vi "Test App Prefix Update is Propagated to Owned Processes.vi"(8 "error in (no error)":errorcluster, 11 "Application Test in":refnum<class "Application Test.lvclass">) -> (0 "error out":errorcluster, 3 "Application Test out":refnum<class "Application Test.lvclass">)   [LabVIEW 2020, in "Application Test.lvclass"]
uses:
  Application Test.lvclass
  Framework/Application/Application.lvclass
  <vilib>/Asteme/LUnit/Test Case.lvclass
  Support/Framework Test Support.lvlib
  Framework/Process/Process.lvclass
  C:/Users/anton/Documents/GitHub/Triarc-Framework/source/Framework/Process/Process.lvclass
  C:/Users/anton/Documents/GitHub/Triarc-Framework/source/Framework/Base/Base.lvclass
  C:/Users/anton/Documents/GitHub/Triarc-Framework/source/Framework/Configuration File/Configuration File.lvclass
  C:/Users/anton/Documents/GitHub/Triarc-Framework/source/Framework/Error Handler Interface/Error Handler Interface.lvclass
  C:/Users/anton/Documents/GitHub/Triarc-Framework/source/Framework/Application/Application.lvclass
  C:/Users/anton/Documents/GitHub/Triarc-Framework/source/Framework Test/Process Test/Process Test.lvclass
  C:/Users/anton/Documents/GitHub/Triarc-Framework/source/Framework Test/Base Class Test/Base Test.lvclass
  C:/Program Files (x86)/National Instruments/LabVIEW 2020/vi.lib/Asteme/LUnit/Test Case.lvclass
  C:/Users/anton/Documents/GitHub/Triarc-Framework/source/Framework Test/Application Test/Application Test.lvclass
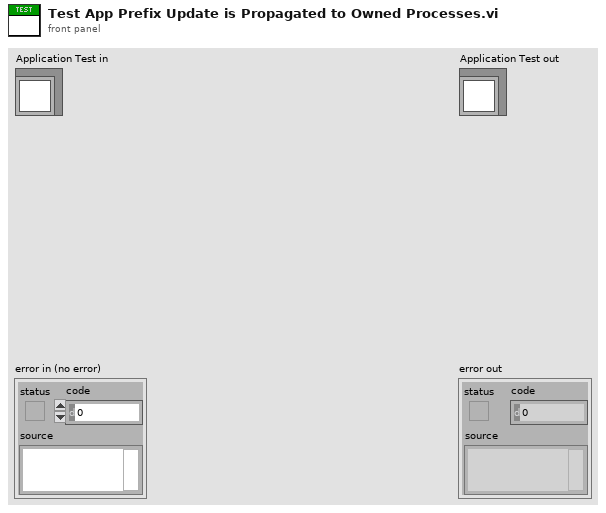
[diagram p1: front panel]
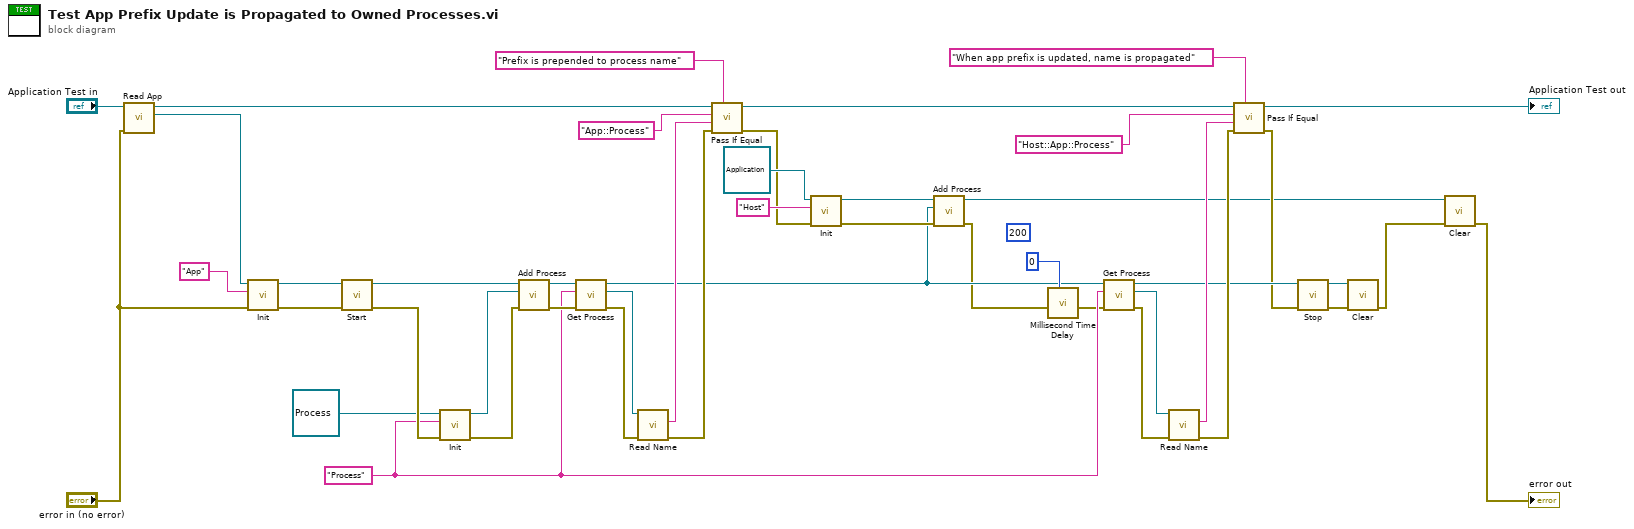
[diagram p0: block diagram]
diagram:
  (unwired) u32 200 ("milliseconds to wait")
  w21 = "Process" ("Name")
  n1 = call "Read App.vi"("error in (no error)"="error in (no error)", "Application Test In"="Application Test in") -> ("App out"=w12:refnum<class "Application.lvclass">, "Application Test Out"=w44:refnum<class "Application Test.lvclass">)  [unwired: 7 in, 1 out]
  n2 = call-dynamic "Init.vi"("error in (no error)"="error in (no error)", "Name"="App", "Process In"=w12) -> ("error out"=w41:errorcluster, "Process Out"=w42:refnum<class "Application.lvclass">)  [unwired: 7 in]
  n3 = call "Start.vi"("error in (no error)"=w41, "Process In"=w42) -> ("error out"=w32:errorcluster, "Process Out"=w40:refnum<class "Application.lvclass">)  [unwired: 8 in]
  n4 = call-dynamic "Init.vi"("error in (no error)"=w32, "Name"=w21, "Process In"=refnum<class "Process.lvclass"> refnum) -> ("error out"=w31:errorcluster, "Process Out"=w36:refnum<class "Process.lvclass">)  [unwired: 7 in]
  n5 = call "Add Process.vi"("error in (no error)"=w31, "Process"=w36, "Rig In"=w40) -> ("error out"=w35:errorcluster, "Rig Out"=w39:refnum<class "Application.lvclass">)  [unwired: 7 in]
  n6 = call "Get Process.vi"("error in (no error)"=w35, "Process Name"=w21, "Rig In"=w39) -> ("error out"=w29:errorcluster, "App Process"=w30:refnum<class "Process.lvclass">, "Rig Out"=w4:refnum<class "Application.lvclass">)  [unwired: 6 in]
  n7 = call-dynamic "Read Name.vi"("error in (no error)"=w29, "Process In"=w30) -> ("error out"=w28:errorcluster, "Qualified Name"=w27:string)  [unwired: 6 in, 2 out]
  n8 = call <vilib>:"Pass If Equal.vi"("Description"="Prefix is prepended to process name", "error in (no error)"=w28, "Actual"=w27, "Expected"="App::Process", "Test Case In"=w44) -> ("error out"=w9:errorcluster, "Test Case Out"=w34:refnum<class "Application Test.lvclass">)  [unwired: 5 in]
  n9 = call-dynamic "Init.vi"("error in (no error)"=w9, "Name"="Host" ("Prefix"), "Process In"=refnum<class "Application.lvclass"> refnum ("Rig In")) -> ("error out"=w7:errorcluster, "Process Out"=w8:refnum<class "Application.lvclass">)  [unwired: 7 in]
  n10 = call "Add Process.vi"("error in (no error)"=w7, "Process"=w4, "Rig In"=w8) -> ("error out"=w3:errorcluster, "Rig Out"=w6:refnum<class "Application.lvclass">)  [unwired: 7 in]
  n11 = call "Millisecond Time Delay.vi"("milliseconds to wait"=u32 0, "error in (no error)"=w3) -> ("error out"=w17:errorcluster)  [unwired: 7 in]
  n12 = call "Get Process.vi"("error in (no error)"=w17, "Process Name"=w21, "Rig In"=w4) -> ("error out"=w23:errorcluster, "App Process"=w24:refnum<class "Process.lvclass">, "Rig Out"=w14:refnum<class "Application.lvclass">)  [unwired: 6 in]
  n13 = call-dynamic "Read Name.vi"("error in (no error)"=w23, "Process In"=w24) -> ("error out"=w18:errorcluster, "Qualified Name"=w22:string)  [unwired: 6 in, 2 out]
  n14 = call <vilib>:"Pass If Equal.vi"("Description"="When app prefix is updated, name is propagated", "error in (no error)"=w18, "Actual"=w22, "Expected"="Host::App::Process", "Test Case In"=w34) -> ("error out"=w13:errorcluster, "Test Case Out"=→"Application Test out":refnum<class "Application Test.lvclass">)  [unwired: 5 in]
  n15 = call "Stop.vi"("error in (no error)"=w13, "Process In"=w14) -> ("error out"=w37:errorcluster, "Process Out"=w38:refnum<class "Application.lvclass">)  [unwired: 7 in, 1 out]
  n16 = call-dynamic "Clear.vi"("error in (no error)"=w37, "Application In"=w38) -> ("error out"=w2:errorcluster)  [unwired: 8 in, 1 out]
  n17 = call-dynamic "Clear.vi"("error in (no error)"=w2, "Application In"=w6) -> ("error out"=→"error out":errorcluster)  [unwired: 8 in, 1 out]
